vi "NHR 9200.vi"() -> ()   [LabVIEW 2018]
uses:
  <instrlib>/niScope/Acquire/niScope Multi Read WDT.vi
  <instrlib>/NHRDCPowerModule/NHRDCPowerModule/NHRDCPowerModule.lvlib
panel:
  out "dt":dbl=10000000.0 min=1.0 max=10000000.0 format="%_3ps"
  in  "Scope Rate":dbl=10000000.0 min=1.0 max=10000000.0 format="%_3pS/s"
  in  "Run Test":bool
  out "Waveform Chart":waveform(dbl)[](graph)
  out "wfm":waveform(dbl)[](array[waveform])
  out "NHR Error":string
  out "Scope On":bool
  out "NHR On":bool
  in  "Current Target":sgl[unit] min=0 max=40
  in  "Voltage":T1={"Ramp Rate (+)"=0.1, "Ramp Rate (-)"=0.1, "Max"=0.0} {"Max" min=0 max=600; "Ramp Rate (+)" min=0.1 max=600; "Ramp Rate (-)" min=0.1}
  out "Stop VI?":bool
  in  "Stop VI":bool
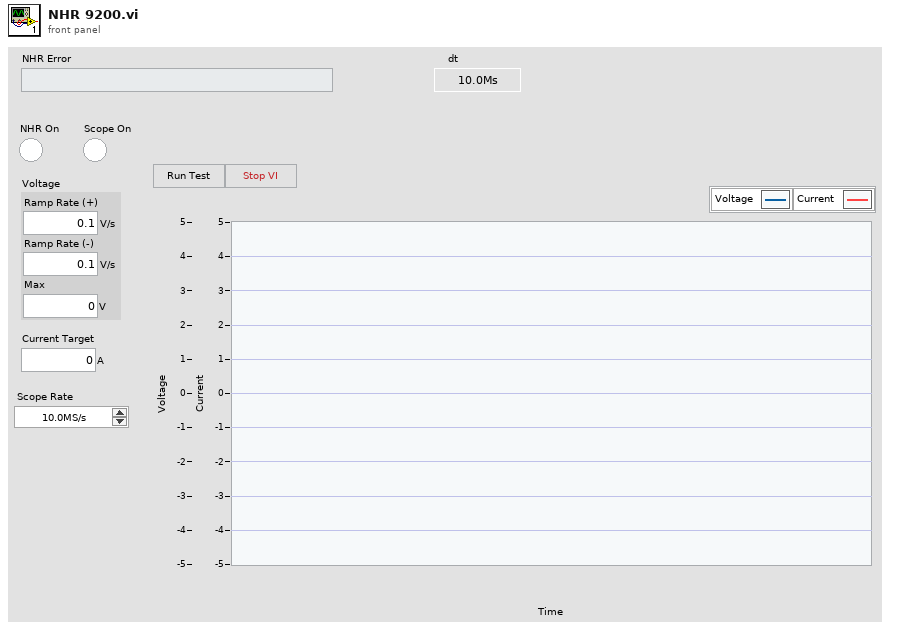
[diagram p1: front panel]
types:
  T1 = cluster{"Ramp Rate (+)":sgl[unit], "Ramp Rate (-)":sgl[unit], "Max":sgl[unit]}
  T2 = enum16{"open", "open or create", "create or replace", "create", "open (read-only)"}
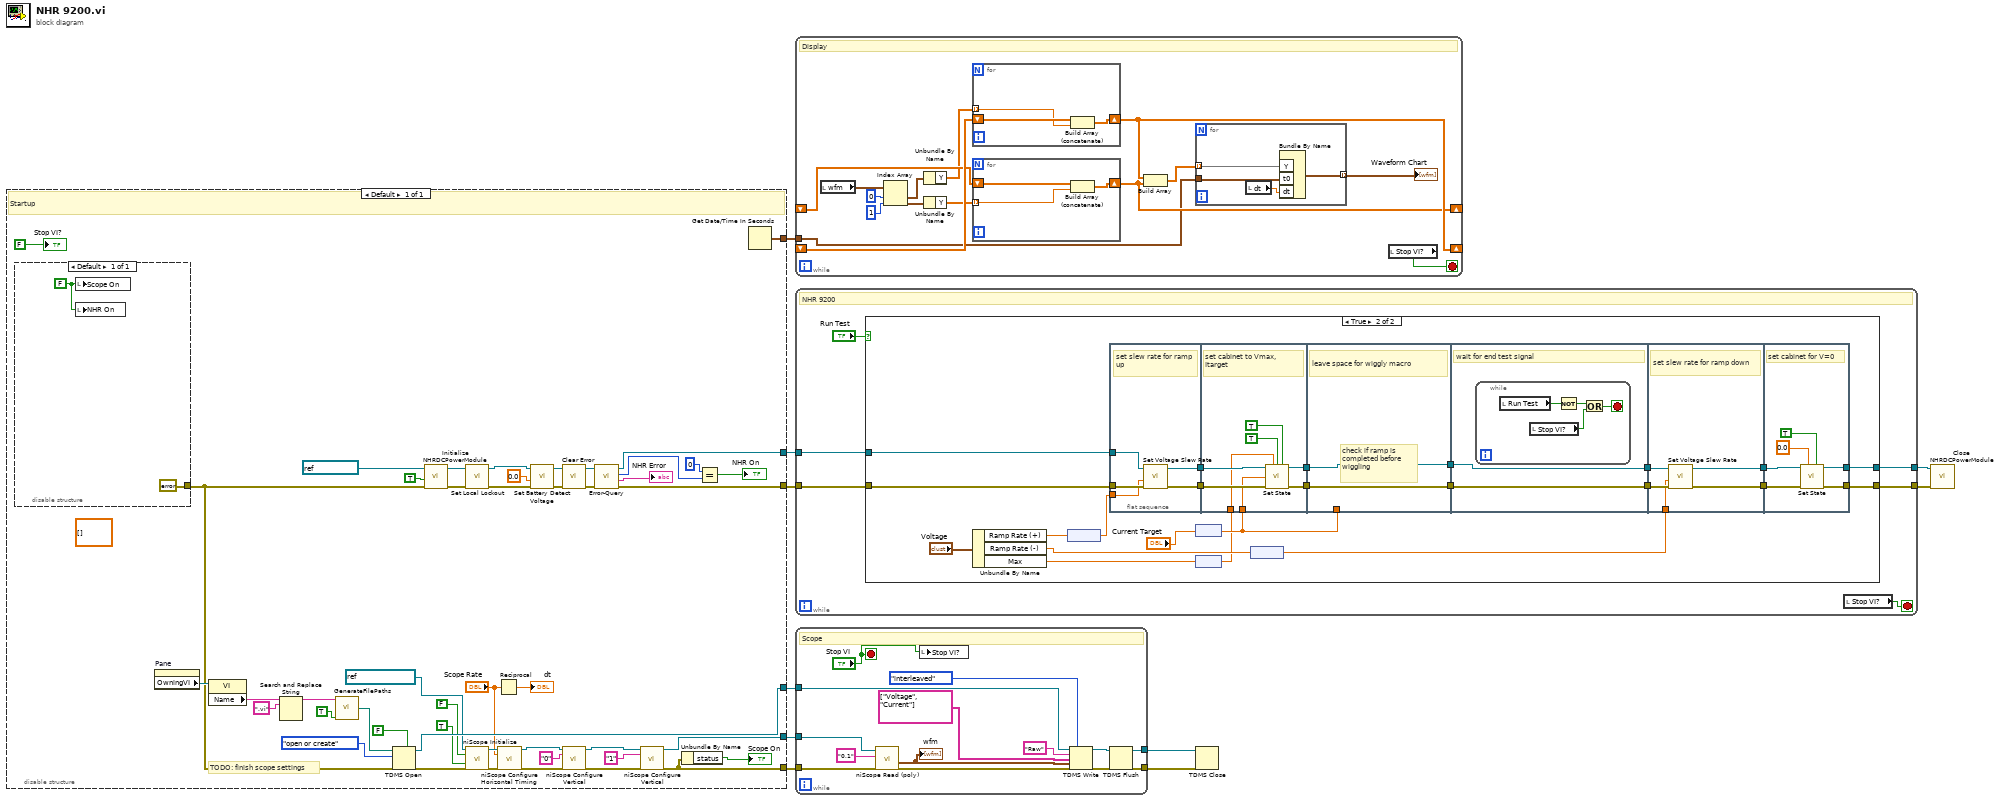
[diagram p0: block diagram]
diagram:
  n1 = disable-structure shown="Default" {
    disable-tunnel: [w56] -> w4
    disable-tunnel: [w44] -> w10
    disable-tunnel: [w22] -> w9
    disable-tunnel: [w37] -> w8
    disable-tunnel: [w36] -> w7
    disable-tunnel: [w17] -> w1
    frame Enabled {
      (unwired) dbl[][] [] ("History Data")
      # "TODO: finish scope settings"
      # "Startup"
      n2 = disable-structure shown="Default" {
        disable-tunnel: [errorcluster {"status"=FALSE, "code"=0, "source"=""} ("error in (no error)")] -> w19
        frame Enabled {
          w58 = FALSE
          n3 = local write "Scope On"(w58) -> ()
          n4 = local write "NHR On"(w58) -> ()
        }
      }
      n5 = property on="Pane" class="Pane"() -> ("OwningVI"=w55:refnum<vi>)  [unwired: 2 in, 2 out]
      n6 = property class="VI"(reference=w55) -> ("Name"=w52:string)  [unwired: 1 in, 2 out]
      n7 = Search and Replace String(input string=w52, search string=".vi") -> (result string=w53:string)  [unwired: 6 in, 3 out]
      n8 = call "GenerateFilePaths.vi"("Logfile? (F)"=TRUE, "Device Name"=w53) -> ("Path"=w28:path)  [unwired: 2 in]
      n9 = TDMS Open(5:FALSE ("create index file? (T)"), 8:w19, 10:T2."open or create" ("operation (0:open)"), 11:w28) -> (0:w30:errorcluster, 3:w56:refnum<k34>)  [unwired: 3 in]
      n10 = call <instrlib>:"Initialize NHRDCPowerModule.vi"("error in (no error)"=w19, "reset device (Off)"=TRUE, "resource name"=refnum<visa-resource-name> "DC PM 1") -> ("error out"=w42:errorcluster, "instrument handle out"=w41:refnum<visa-resource-name>)  [unwired: 7 in]
      n11 = call <instrlib>:"Set Local Lockout.vi"("error in (no error)"=w42, "instrument handle"=w41) -> ("error out"=w35:errorcluster, "instrument handle out"=w33:refnum<visa-resource-name>)  [unwired: 8 in]
      n12 = call <instrlib>:"niScope Initialize.vi"("resource name"=refnum<k15> "oscilloscope", "id query"=FALSE, "reset device"=TRUE, "error in"=w30) -> ("instrument handle"=w15:refnum<k15>, "error out"=w14:errorcluster)  [unwired: 10 in]
      n13 = Reciprocal(x="Scope Rate") -> (1/x=→"dt":dbl)
      n14 = call <instrlib>:"niScope Configure Horizontal Timing.vi"("instrument handle"=w15, "min sample rate"="Scope Rate", "error in"=w14) -> ("instrument handle out"=w16:refnum<k15>, "error out"=w13:errorcluster)  [unwired: 11 in]
      n15 = call <instrlib>:"Set Battery Detect Voltage.vi"("error in (no error)"=w35, "minimum voltage (4.0)"=sgl 0.0, "instrument handle"=w33) -> ("error out"=w34:errorcluster, "instrument handle out"=w32:refnum<visa-resource-name>)  [unwired: 7 in]
      n16 = call <instrlib>:"Clear Error.vi"("error in (no error)"=w34, "instrument handle"=w32) -> ("error out"=w39:errorcluster, "instrument handle out"=w38:refnum<visa-resource-name>)  [unwired: 8 in]
      n17 = call <instrlib>:"niScope Configure Vertical.vi"("instrument handle"=w16, "channels"="0", "error in"=w13) -> ("instrument handle out"=w46:refnum<k15>, "error out"=w45:errorcluster)  [unwired: 11 in]
      n18 = call <instrlib>:"Error-Query.vi"("error in (no error)"=w39, "instrument handle"=w38) -> ("error out"=w37:errorcluster, "error message"=→"NHR Error":string, "error code"=w25:i32, "instrument handle out"=w36:refnum<visa-resource-name>)  [unwired: 6 in]
      n19 = call <instrlib>:"niScope Configure Vertical.vi"("instrument handle"=w46, "channels"="1", "error in"=w45) -> ("instrument handle out"=w44:refnum<k15>, "error out"=w22:errorcluster)  [unwired: 11 in]
      n20 = Unbundle By Name(w22) -> ("status"=→"Scope On":bool)
      n21 = Equal?(x=0, y=w25) -> (x = y?=→"NHR On":bool)
      n22 = Get Date/Time In Seconds() -> (seconds since 1Jan1904=w17:timestamp)
      "Stop VI?" <- FALSE
    }
  }
  n23 = while {
    shift-right: [w64] -> _
    shift-left: _ -> [w72]
    shift-right: [w63] -> _
    shift-left: _ -> [w67]
    tunnel: w1 -> [w61]
    stop <- w73 stop-if-true
    # "Display"
    n24 = local read "wfm"() -> (w62:waveform(dbl)[])
    n25 = Index Array(array=w62, index #1=0 ("index"), index #2=1 ("index")) -> (element #1=w71:waveform(dbl), element #2=w70:waveform(dbl))
    n26 = Unbundle By Name(w71) -> ("Y"=w65:dbl[])
    n27 = Unbundle By Name(w70) -> ("Y"=w66:dbl[])
    n28 = for {
      tunnel: w65 -> [w81] mode=indexing
      shift-right: [w82] -> w64
      shift-left: w72 -> [w83]
      n29 = Build Array (concatenate)(w83, w81) -> (w82:dbl[])
    }
    n30 = for {
      tunnel: w66 -> [w79] mode=indexing
      shift-right: [w78] -> w63
      shift-left: w67 -> [w80]
      n31 = Build Array (concatenate)(w80, w79) -> (w78:dbl[])
    }
    n32 = Build Array(w64, w63) -> (w60:dbl[][])
    n33 = for {
      tunnel: w61 -> [w77]
      tunnel: w60 -> [w75] mode=indexing
      tunnel: [w74] -> w59 mode=indexing
      n34 = local read "dt"() -> (w76:dbl)
      n35 = Bundle By Name("Y"=w75, "t0"=w77, "dt"=w76) -> (w74:waveform(dbl))  [unwired: 1 in]
    }
    "Waveform Chart" <- w59
    n36 = local read "Stop VI?"() -> (w73:bool)
  }
  n37 = while {
    tunnel: w8 -> [w88]
    tunnel: w7 -> [w89]
    tunnel: [w85] -> w6
    tunnel: [w84] -> w5
    stop <- w86 stop-if-true
    # "NHR 9200"
    n38 = case shown="True" "Run Test" {
      tunnel: w89 -> [w90 w108]
      tunnel: w88 -> [w91 w107]
      tunnel: [w90 w93] -> w85
      tunnel: [w91 w92] -> w84
      frame False {
      }
      frame True {
        n39 = Unbundle By Name("Voltage") -> ("Ramp Rate (+)"=w105:sgl[unit], "Ramp Rate (-)"=w109:sgl[unit], "Max"=w111:sgl[unit])
        n40 = node(w105) -> (w104:sgl)
        n41 = flat-sequence {
          tunnel: w108 -> [w119]
          tunnel: w107 -> [w118]
          tunnel: [w117] -> w114
          tunnel: [w116] -> w113
          tunnel: w104 -> [w115]
          tunnel: w102 -> [w124]
          tunnel: w106 -> [w125]
          tunnel: w114 -> [w127]
          tunnel: w113 -> [w126]
          tunnel: [w121] -> w99
          tunnel: [w120] -> w96
          tunnel: [w129] -> w100
          tunnel: [w128] -> w97
          tunnel: w96 -> [w128]
          tunnel: w99 -> [w129]
          tunnel: w106 -> [_]
          tunnel: [w131] -> w101
          tunnel: w100 -> [w131]
          tunnel: [w130] -> w98
          tunnel: w97 -> [w130]
          tunnel: w103 -> [w138]
          tunnel: w101 -> [w140]
          tunnel: w98 -> [w139]
          tunnel: [w137] -> w95
          tunnel: [w136] -> w94
          tunnel: w95 -> [w146]
          tunnel: w94 -> [w145]
          tunnel: [w142] -> w93
          tunnel: [w141] -> w92
          frame #0 {
            # "set slew rate for ramp up"
            n42 = call <instrlib>:"Set Voltage Slew Rate.vi"("error in (no error)"=w118, "voltage slew rate (0.0)"=w115, "instrument handle"=w119) -> ("error out"=w116:errorcluster, "instrument handle out"=w117:refnum<visa-resource-name>)  [unwired: 7 in]
          }
          frame #1 {
            # "set cabinet to Vmax, Itarget"
            n43 = call <instrlib>:"Set State.vi"("instrument handle"=w127, "voltage (0.0)"=w124, "current enabled (false)"=TRUE, "voltage enabled (false)"=TRUE, "current (0.0)"=w125, "error in (no error)"=w126) -> ("instrument handle out"=w121:refnum<visa-resource-name>, "error out"=w120:errorcluster)  [unwired: 8 in]
          }
          frame #2 {
            # "check if ramp is completed before wiggling"
            # "leave space for wiggly macro"
          }
          frame #3 {
            # "wait for end test signal"
            n44 = while {
              stop <- w132 stop-if-true
              n45 = local read "Run Test"() -> (w135:bool)
              n46 = local read "Stop VI?"() -> (w133:bool)
              n47 = Not(x=w135) -> (.not. x?=w134:bool)
              n48 = Or(x=w134, y=w133) -> (x .or. y?=w132:bool)
            }
          }
          frame #4 {
            # "set slew rate for ramp down"
            n49 = call <instrlib>:"Set Voltage Slew Rate.vi"("error in (no error)"=w139, "voltage slew rate (0.0)"=w138, "instrument handle"=w140) -> ("error out"=w137:errorcluster, "instrument handle out"=w136:refnum<visa-resource-name>)  [unwired: 7 in]
          }
          frame #5 {
            # "set cabinet for V=0"
            n50 = call <instrlib>:"Set State.vi"("instrument handle"=w145, "voltage (0.0)"=sgl 0.0, "voltage enabled (false)"=TRUE, "error in (no error)"=w146) -> ("instrument handle out"=w142:refnum<visa-resource-name>, "error out"=w141:errorcluster)  [unwired: 10 in]
          }
        }
        n51 = node("Current Target") -> (w106:sgl)
        n52 = node(w111) -> (w102:sgl)
        n53 = node(w109) -> (w103:sgl)
      }
    }
    n54 = local read "Stop VI?"() -> (w86:bool)
  }
  n55 = while {
    tunnel: w10 -> [w159]
    tunnel: w9 -> [w158]
    tunnel: w4 -> [w152]
    tunnel: [w148] -> w3
    tunnel: [w147] -> w2
    stop <- "Stop VI" stop-if-true
    # "Scope"
    n56 = call-poly <instrlib>:"niScope Read (poly).vi"("error in"=w158, "channels"="0,1", "instrument handle"=w159) -> ("error out"=w154:errorcluster, "wfm"=w153:waveform(dbl)[])  [unwired: 5 in, 2 out]
    "wfm" <- w153
    n57 = local write "Stop VI?"("Stop VI") -> ()
    n58 = TDMS Write(0:w152, 1:enum16{"decimated", "interleaved"}."interleaved" ("data layout (0:decimated)"), 5:"Raw" ("group name in (Untitled)"), 7:string[] ["Voltage", "Current"] ("channel name(s) in (Untitled)"), 9:w153, 11:w154) -> (4:w150:refnum<k34>, 15:w149:errorcluster)  [unwired: 2 out]
    n59 = TDMS Flush(4:w149, 7:w150) -> (0:w148:errorcluster, 3:w147:refnum<k34>)
  }
  n60 = TDMS Close(8:w3, 11:w2) -> ()  [unwired: 2 out]
  n61 = call <instrlib>:"Close NHRDCPowerModule.vi"("error in (no error)"=w5, "instrument handle"=w6) -> ()  [unwired: 9 in, 1 out]
